vi "REG - Generate2DTrain.vi"(8 "error in":errorcluster, 11 "Local":T5={"Parameters"={"Plot"=refnum, "Data"={"Split"={"X Train"=[], "X Test"=[], "Y Train"=[], "Y Test"=[]}, "Predict"=[]}, "Display"={"Choice"=enum."All", "Indexe"={"X"=0, "Y"=1}}, "Point Property"={"Train Style"=enum."Full circle", "Test OK Style"=enum."Full square", "Label Color"=[8978528, 4367871, 16716800], "Test NO OK"={"Style"=enum."Cross", "Color"=16711680}}, "Tolerance's threshold"=0.0}, "2D Array"=[], "Point ID"=[], "GoodPredict"=0, "Rating 2D Array"=[]}) -> (0 "error out":errorcluster, 3 "Local_Out":T5={"Parameters"={"Plot"=refnum, "Data"={"Split"={"X Train"=[], "X Test"=[], "Y Train"=[], "Y Test"=[]}, "Predict"=[]}, "Display"={"Choice"=enum."All", "Indexe"={"X"=0, "Y"=0}}, "Point Property"={"Train Style"=enum."Full circle", "Test OK Style"=enum."Full square", "Label Color"=[8978528, 4367871, 16716800], "Test NO OK"={"Style"=enum."Cross", "Color"=16711680}}, "Tolerance's threshold"=0.0}, "2D Array"=[], "Point ID"=[], "GoodPredict"=0, "Rating 2D Array"=[]})   [LabVIEW 2020]
doc: "Generate 2D graph"
uses:
  _Controls/Datas.ctl
  _Controls/PointPropertyMultipleLabel.ctl
  _Controls/Style.ctl
  _Controls/2DData.ctl
types:
  T1 = typedef "Datas.ctl" = cluster{"Split":cluster{"X Train":dbl[][], "X Test":dbl[][], "Y Train":dbl[][], "Y Test":dbl[][]}, "Predict":dbl[][]}
  T2 = typedef "PointPropertyMultipleLabel.ctl" = cluster{"Train Style":T3, "Test OK Style":T3, "Label Color":u32[], "Test NO OK":cluster{"Style":T3, "Color":u32}}
  T3 = typedef "Style.ctl" = enum16{"Empty circle", "Full circle", "Empty square", "Full square", "Cross"}
  T4 = typedef "2DData.ctl" = cluster{"Tag":i32, "X":dbl[], "Y":dbl[]}
  T5 = cluster{"Parameters":cluster{"Plot":refnum<vi>, "Data":T1, "Display":cluster{"Choice":enum16{"All", "Train", "Test"}, "Indexe":cluster{"X":i32, "Y":i32}}, "Point Property":T2, "Tolerance's threshold":dbl}, "2D Array":cluster{"X":dbl[], "Y":dbl[]}[], "Point ID":cluster{"DataUse":enum16{"Dataset", "Train", "Test"}, "Color":u32}[], "GoodPredict":i32, "Rating 2D Array":T4[]}
  T6 = cluster{"DataUse":enum16{"Dataset", "Train", "Test"}, "Color":u32}
  T7 = cluster{"X Train":dbl[][], "X Test":dbl[][], "Y Train":dbl[][], "Y Test":dbl[][]}
  T8 = cluster{"DataUse":enum16{"Dataset", "Train", "Test"}, "Color":u32}[]
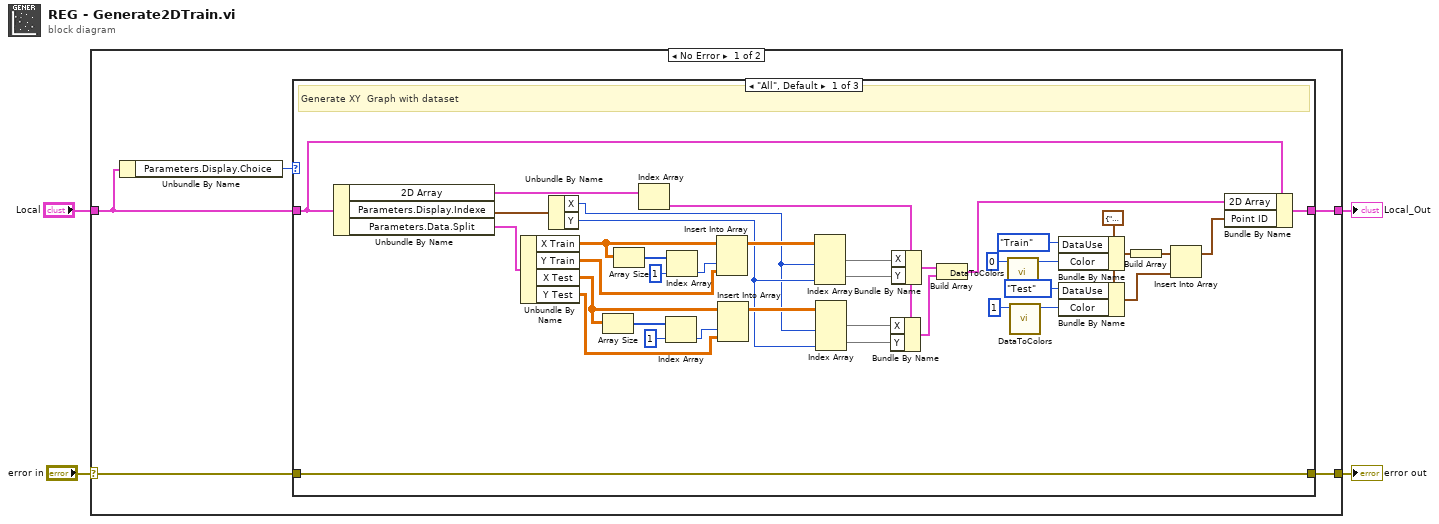
[diagram p0: block diagram]
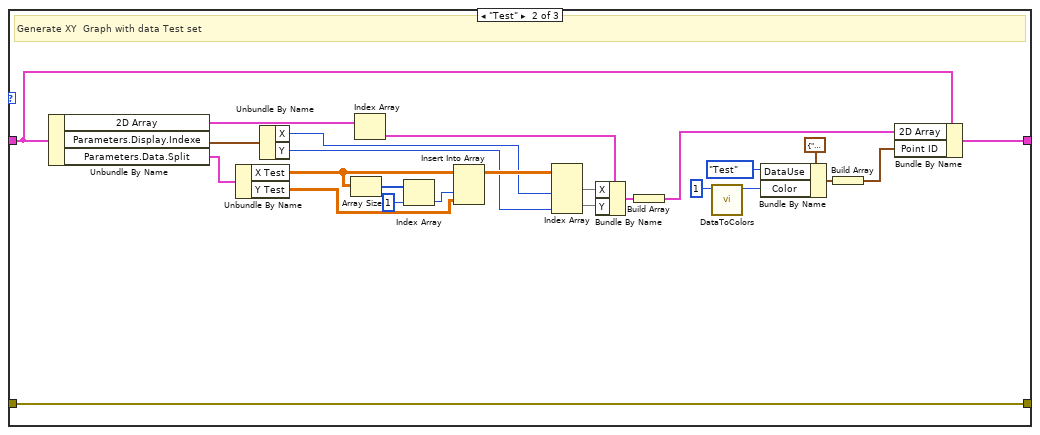
[diagram p2: hidden frame]
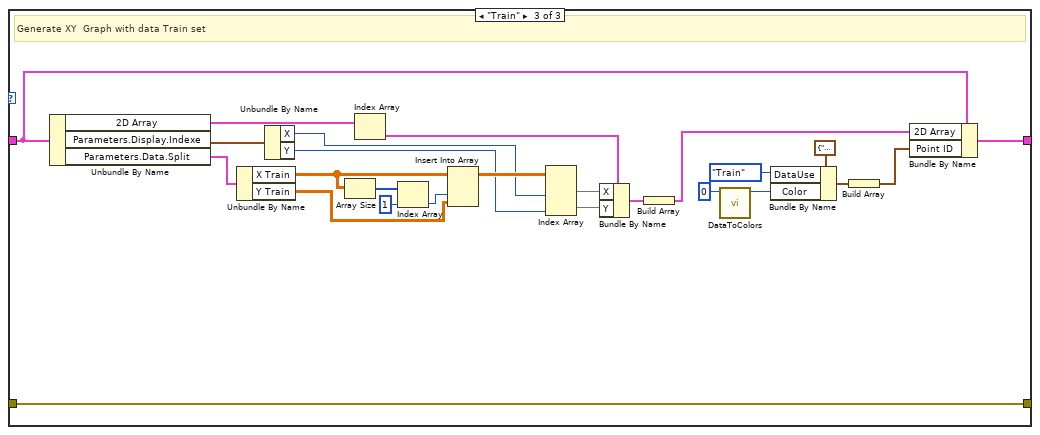
[diagram p3: hidden frame]
diagram:
  n1 = case shown="No Error" "error in" {
    selector: "error in" -> [w7 w99]
    tunnel: "Local" -> [w8 w100]
    tunnel: [w6 w100] -> w1
    tunnel: [w5 w99] -> w3
    frame No Error {
      n2 = Unbundle By Name(w8) -> ("Parameters.Display.Choice"=w9:enum16{"All", "Train", "Test"})
      n3 = case shown="\"All\", Default" w9 {
        tunnel: w7 -> [w42 w69 w94]
        tunnel: w8 -> [w47 w72 w97]
        tunnel: [w46 w71 w96] -> w6
        tunnel: [w42 w69 w94] -> w5
        frame "All", Default {
          w30 = T6 {"DataUse"=enum."Train", "Color"=0}
          # "Generate XY  Graph with dataset"
          n4 = Unbundle By Name(w47) -> ("2D Array"=w35:cluster{"X":dbl[], "Y":dbl[]}[], "Parameters.Display.Indexe"=w43:cluster{"X":i32, "Y":i32}, "Parameters.Data.Split"=w48:T7)
          n5 = Unbundle By Name(w48) -> ("X Train"=w20:dbl[][], "Y Train"=w29:dbl[][], "X Test"=w15:dbl[][], "Y Test"=w23:dbl[][])
          n6 = Unbundle By Name(w43) -> ("X"=w12:i32, "Y"=w24:i32)
          n7 = Array Size(array=w15) -> (size(s)=w16:i32[])
          n8 = Array Size(array=w20) -> (size(s)=w19:i32[])
          n9 = Index Array(array=w35) -> (element=w34:cluster{"X":dbl[], "Y":dbl[]})  [unwired: 1 in]
          n10 = Index Array(array=w16, index=1) -> (element=w14:i32)
          n11 = Index Array(array=w19, index=1) -> (element=w17:i32)
          n12 = Insert Into Array(array=w20, index (col)=w17, new element=w29) -> (w28:dbl[][])  [unwired: 1 in]
          n13 = Insert Into Array(array=w15, index (col)=w14, new element=w23) -> (w25:dbl[][])  [unwired: 1 in]
          n14 = Index Array(array=w28, index (col) #1=w12, index (col) #2=w24) -> (element #1=w27:dbl[], element #2=w26:dbl[])  [unwired: 2 in]
          n15 = Index Array(array=w25, index (col) #1=w12, index (col) #2=w24) -> (element #1=w22:dbl[], element #2=w21:dbl[])  [unwired: 2 in]
          n16 = Bundle By Name(cluster=w34, "X"=w22, "Y"=w21) -> (w11:cluster{"X":dbl[], "Y":dbl[]})
          n17 = Bundle By Name(cluster=w34, "X"=w27, "Y"=w26) -> (w10:cluster{"X":dbl[], "Y":dbl[]})
          n18 = Build Array(w10, w11) -> (w33:cluster{"X":dbl[], "Y":dbl[]}[])
          n19 = call "DataToColors.vi"("Label"=0) -> ("Color"=w41:u32)  [unwired: 10 in]
          n20 = call "DataToColors.vi"("Label"=1) -> ("Color"=w39:u32)  [unwired: 10 in]
          n21 = Bundle By Name(cluster=w30, "DataUse"=enum16{"Dataset", "Train", "Test"}."Train", "Color"=w41) -> (w32:T6)
          n22 = Bundle By Name(cluster=w30, "DataUse"=enum16{"Dataset", "Train", "Test"}."Test", "Color"=w39) -> (w45:T6)
          n23 = Build Array(w32) -> (w31:T8)
          n24 = Insert Into Array(array=w31, new element=w45) -> (w44:T8)  [unwired: 1 in]
          n25 = Bundle By Name(cluster=w47, "2D Array"=w33, "Point ID"=w44) -> (w46:T5)
        }
        frame "Test" {
          # "Generate XY  Graph with data Test set"
          n26 = Unbundle By Name(w72) -> ("2D Array"=w65:cluster{"X":dbl[], "Y":dbl[]}[], "Parameters.Display.Indexe"=w70:cluster{"X":i32, "Y":i32}, "Parameters.Data.Split"=w73:T7)
          n27 = Unbundle By Name(w73) -> ("X Test"=w54:dbl[][], "Y Test"=w53:dbl[][])
          n28 = Unbundle By Name(w70) -> ("X"=w52:i32, "Y"=w51:i32)
          n29 = Array Size(array=w54) -> (size(s)=w57:i32[])
          n30 = Index Array(array=w65) -> (element=w64:cluster{"X":dbl[], "Y":dbl[]})  [unwired: 1 in]
          n31 = Index Array(array=w57, index=1) -> (element=w55:i32)
          n32 = Insert Into Array(array=w54, index (col)=w55, new element=w53) -> (w58:dbl[][])  [unwired: 1 in]
          n33 = Index Array(array=w58, index (col) #1=w52, index (col) #2=w51) -> (element #1=w50:dbl[], element #2=w49:dbl[])  [unwired: 2 in]
          n34 = Bundle By Name(cluster=w64, "X"=w50, "Y"=w49) -> (w63:cluster{"X":dbl[], "Y":dbl[]})
          n35 = Build Array(w63) -> (w62:cluster{"X":dbl[], "Y":dbl[]}[])
          n36 = call "DataToColors.vi"("Label"=1) -> ("Color"=w68:u32)  [unwired: 10 in]
          n37 = Bundle By Name(cluster=T6 {"DataUse"=enum."Train", "Color"=0}, "DataUse"=enum16{"Dataset", "Train", "Test"}."Test", "Color"=w68) -> (w60:T6)
          n38 = Build Array(w60) -> (w59:T8)
          n39 = Bundle By Name(cluster=w72, "2D Array"=w62, "Point ID"=w59) -> (w71:T5)
        }
        frame "Train" {
          # "Generate XY  Graph with data Train set"
          n40 = Unbundle By Name(w97) -> ("2D Array"=w90:cluster{"X":dbl[], "Y":dbl[]}[], "Parameters.Display.Indexe"=w95:cluster{"X":i32, "Y":i32}, "Parameters.Data.Split"=w98:T7)
          n41 = Unbundle By Name(w98) -> ("X Train"=w79:dbl[][], "Y Train"=w78:dbl[][])
          n42 = Unbundle By Name(w95) -> ("X"=w77:i32, "Y"=w76:i32)
          n43 = Array Size(array=w79) -> (size(s)=w82:i32[])
          n44 = Index Array(array=w90) -> (element=w89:cluster{"X":dbl[], "Y":dbl[]})  [unwired: 1 in]
          n45 = Index Array(array=w82, index=1) -> (element=w80:i32)
          n46 = Insert Into Array(array=w79, index (col)=w80, new element=w78) -> (w83:dbl[][])  [unwired: 1 in]
          n47 = Index Array(array=w83, index (col) #1=w77, index (col) #2=w76) -> (element #1=w75:dbl[], element #2=w74:dbl[])  [unwired: 2 in]
          n48 = Bundle By Name(cluster=w89, "X"=w75, "Y"=w74) -> (w88:cluster{"X":dbl[], "Y":dbl[]})
          n49 = Build Array(w88) -> (w87:cluster{"X":dbl[], "Y":dbl[]}[])
          n50 = call "DataToColors.vi"("Label"=0) -> ("Color"=w93:u32)  [unwired: 10 in]
          n51 = Bundle By Name(cluster=T6 {"DataUse"=enum."Train", "Color"=0}, "DataUse"=enum16{"Dataset", "Train", "Test"}."Train", "Color"=w93) -> (w86:T6)
          n52 = Build Array(w86) -> (w84:T8)
          n53 = Bundle By Name(cluster=w97, "2D Array"=w87, "Point ID"=w84) -> (w96:T5)
        }
      }
    }
    frame Error {
    }
  }
  "error out" <- w3
  "Local_Out" <- w1
